vi "Check pre-empt.vi"(8 "error in (no error)":errorcluster, 11 "_Popup in":refnum<class "Popup.lvclass">) -> (0 "error out":errorcluster, 1 "notification":variant, 2 "Pre-empted?":bool)   [LabVIEW 2021, in "Pop-Up.lvlib" / "Popup.lvclass"]
doc: "check on the status of the pre-empt notifier\n\n<b>Code Developed By:</b> +\nDaniel Coons +\nhttps://github.com/danielcoons/tsc-pop-up"
uses:
  Popup.lvclass
  Popup.lvclass/Popup.ctl
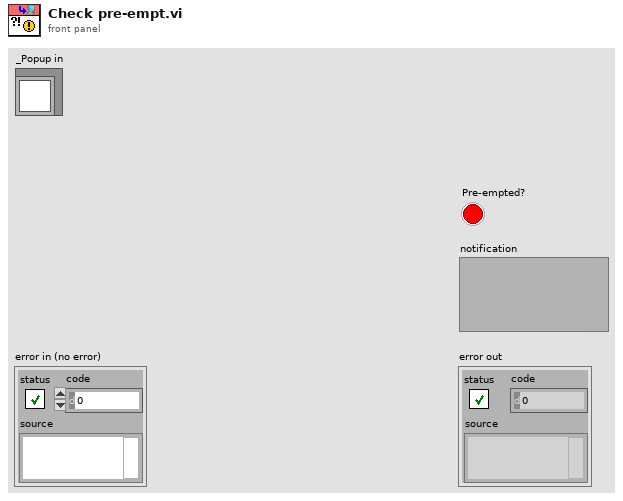
[diagram p1: front panel]
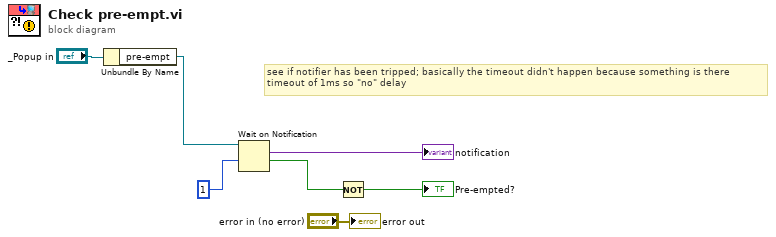
[diagram p0: block diagram]
diagram:
  # "see if notifier has been tripped; basically the timeout didn't happen because something is there\ntimeout of 1ms so \"no\" delay"
  n1 = Unbundle By Name("_Popup in") -> ("pre-empt"=w5:refnum<notifier>)
  n2 = Wait on Notification(notifier=w5, timeout in ms (-1)=1) -> (notification=→"notification":variant, timed out?=w3:bool)  [unwired: 2 in, 2 out]
  n3 = Not(x=w3) -> (.not. x?=→"Pre-empted?":bool)
  "error out" <- "error in (no error)"
